vi "Verify.vi"(8 "error in (no error)":errorcluster, 9 "Role":string, 10 "User":string, 11 "Credentials in":refnum<class "Credentials.lvclass">) -> (0 "error out":errorcluster, 2 "Verified?":bool, 3 "Credentials out":refnum<class "Credentials.lvclass">)   [LabVIEW 2016, in "Credentials.lvclass"]
uses:
  Credentials.lvclass
  Credentials.lvclass/Credentials.ctl
  LUT/LUT.lvclass
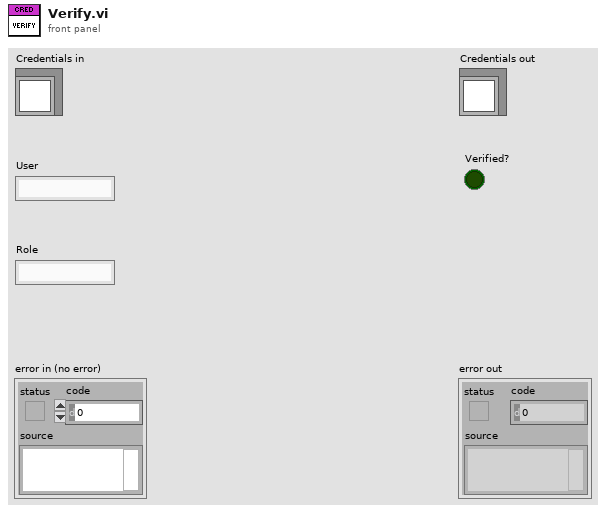
[diagram p1: front panel]
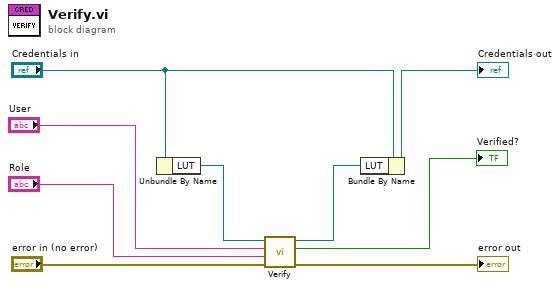
[diagram p0: block diagram]
diagram:
  n1 = Unbundle By Name("Credentials in") -> ("LUT"=w6:refnum<class "LUT.lvclass">)
  n2 = call "Verify.vi"("error in (no error)"="error in (no error)", "Value"="Role", "Key"="User", "LUT in"=w6) -> ("error out"=→"error out":errorcluster, "Verified?"=→"Verified?":bool, "LUT out"=w4:refnum<class "LUT.lvclass">)  [unwired: 5 in]
  n3 = Bundle By Name(cluster="Credentials in", "LUT"=w4) -> (→"Credentials out":refnum<class "Credentials.lvclass">)
